vi "Read Text Width.vi"(9 "Digital in":refnum<class "Digital.lvclass">) -> (3 "Digital out":refnum<class "Digital.lvclass">, 4 "Text Width":u32)   [LabVIEW 2014, in "Digital.lvclass"]
uses:
  Digital.lvclass
  Digital.lvclass/Digital.ctl
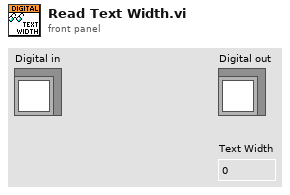
[diagram p1: front panel]
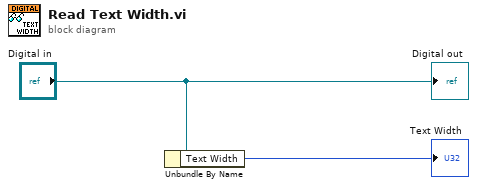
[diagram p0: block diagram]
diagram:
  n1 = Unbundle By Name("Digital in") -> ("Text Width"=→"Text Width":u32)
  "Digital out" <- "Digital in"
